vi "CreatePrivateEvents.vi"(8 "error in (no error)":errorcluster, 11 "Generator":refnum<class "Generator.lvclass">) -> (0 "error out":errorcluster, 3 "Generator out":refnum<class "Generator.lvclass">)   [LabVIEW 2016, in "Generator.lvclass"]
doc: "---------------------------------------------------------------\nJKI State Machine Objects™\nhttp://jki.net/state-machine-objects/\nCopyright (C) 2005-2015, JKI <info@jki.net>\nALL RIGHTS RESERVEDJKI State Machine Objects (SMO) 1.0.0.4\nJKI - JKI\nCopyright (c) 2015, JKI"
uses:
  Generator.lvclass
  Typedefs/PrivateEvents--Generator.configGenerator.ctl
  Typedefs/PrivateEvents--Generator.resetGenerator.ctl
  Typedefs/PrivateEvents--Generator.configSampling.ctl
  Typedefs/PrivateEvents--Generator.askWaveform.ctl
  Generator.lvclass/Generator.ctl
  <vilib>/JKI/JKI SMO/SMO/SMO.lvclass
panel:
  # "For instructions on how to use the JKI State Machine Objects, examples and video tutorials, visit:\nhttp://jki.net/state-machine-objects/\n\nJKI State Machine Objects™\nhttp://jki.net/state-machine-objects/\nCopyright (C) 2005-2015, JKI <info@jki.net>\nALL RIGHTS RESERVED"
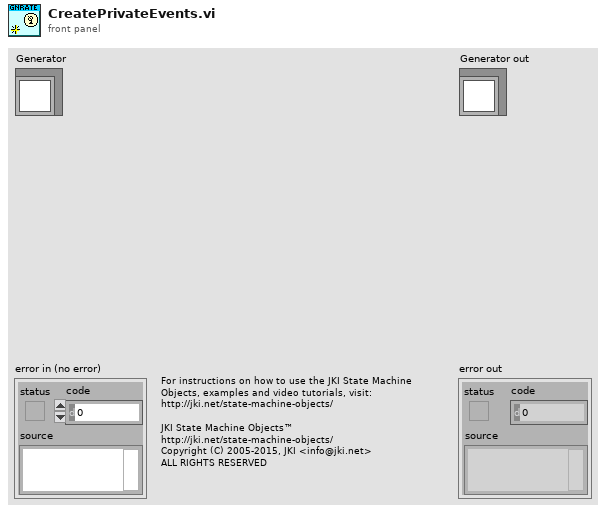
[diagram p1: front panel]
types:
  T1 = typedef "Generator.lvclass/PrivateEvents--Generator.askWaveform.ctl" = string
  T2 = typedef "Generator.lvclass/PrivateEvents--Generator.configSampling.ctl" = cluster{"Fs":dbl, "#s":dbl}
  T3 = typedef "Generator.lvclass/PrivateEvents--Generator.resetGenerator.ctl" = bool
  T4 = typedef "Generator.lvclass/PrivateEvents--Generator.configGenerator.ctl" = cluster{"A (V)":dbl, "DC (V)":dbl, "f (Hz)":dbl, "phi (deg)":dbl, "signal type":enum16{"Sine Wave", "Triangle Wave", "Square Wave", "Sawtooth Wave"}}[]
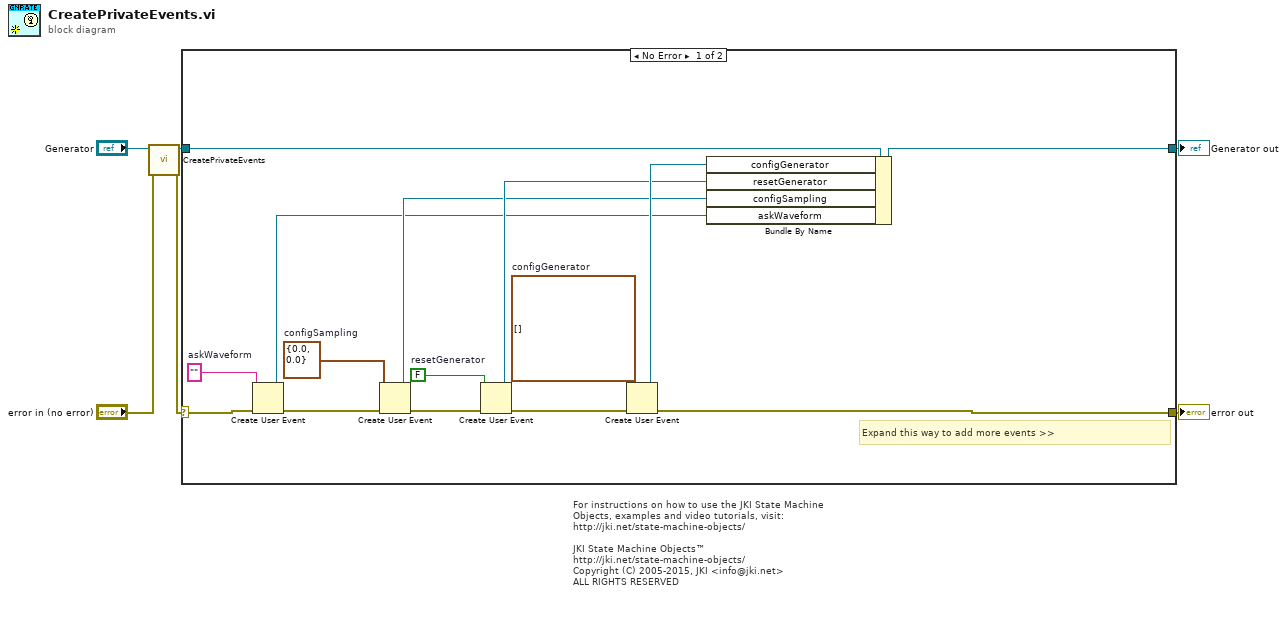
[diagram p0: block diagram]
diagram:
  # "For instructions on how to use the JKI State Machine Objects, examples and video tutorials, visit:\nhttp://jki.net/state-machine-objects/\n\nJKI State Machine Objects™\nhttp://jki.net/state-machine-objects/\nCopyright (C) 2005-2015, JKI <info@jki.net>\nALL RIGHTS RESERVED"
  n1 = call-parent "CreatePrivateEvents.vi"("error in (no error)"="error in (no error)", "SMO"="Generator") -> ("error out"=w1:errorcluster, "SMO out"=w3:refnum<class "Generator.lvclass">)  [unwired: 8 in]
  n2 = case shown="No Error" w1 {
    selector: w1 -> [w20 w23]
    tunnel: [w18 w23] -> w5
    tunnel: [w19 w22] -> w6
    tunnel: w3 -> [w21 w22]
    frame No Error {
      w8 = T1 ""  # askWaveform
      w11 = T2 {"Fs"=0.0, "#s"=0.0}  # configSampling
      w14 = T3 FALSE  # resetGenerator
      w17 = T4 []  # configGenerator
      # "Expand this way to add more events >>"
      n3 = Create User Event(user event datatype=w8, error in=w20) -> (user event=w7:refnum<user-event>, error out=w9:errorcluster)
      n4 = Create User Event(user event datatype=w11, error in=w9) -> (user event=w10:refnum<user-event>, error out=w12:errorcluster)
      n5 = Create User Event(user event datatype=w14, error in=w12) -> (user event=w13:refnum<user-event>, error out=w15:errorcluster)
      n6 = Create User Event(user event datatype=w17, error in=w15) -> (user event=w16:refnum<user-event>, error out=w18:errorcluster)
      n7 = Bundle By Name(cluster=w21, "configGenerator"=w16, "resetGenerator"=w13, "configSampling"=w10, "askWaveform"=w7) -> (w19:refnum<class "Generator.lvclass">)
    }
    frame Error {
    }
  }
  "error out" <- w5
  "Generator out" <- w6
